vi "calculate Psi.vi"(0 "Chi_i":dbl, 11 "a":dbl) -> (8 "Psi_i":dbl)   [LabVIEW 2017, in "LicorLI7000.lvlib"]
uses:
  LicorLI7000.lvlib
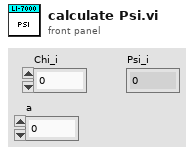
[diagram p1: front panel]
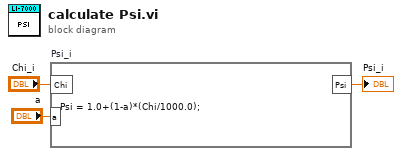
[diagram p0: block diagram]
diagram:
  n1 = formula code="Psi = 1.0+(1-a)*(Chi/1000.0);" "Psi_i"("Chi"="Chi_i", "a"="a") -> ("Psi"=→"Psi_i":dbl)
